vi "Tosca-Clear Trial Marker.vi"(11 "AODO":T1) -> (3 "AODO Out":T1)   [LabVIEW 2020]
uses:
  Typedefs/Tosca-State AODO.ctl
  epl-vi-lib/Signal Synthesis VIs/4th Generation/Classes/SignalManager/SignalManager.lvclass
  Typedefs/Tosca-AO Runtime.ctl
  Typedefs/Tosca-DO Runtime.ctl
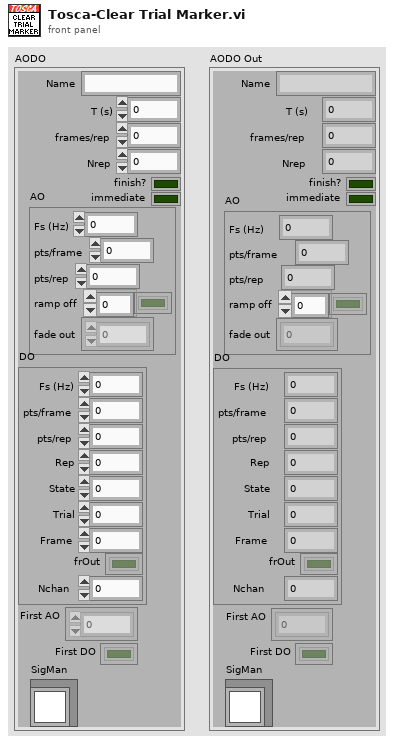
[diagram p1: front panel]
types:
  T1 = typedef "Tosca-State AODO.ctl" = cluster{"Name":string, "T (s)":dbl, "First AO":dbl[][], "frames/rep":i32, "finish?":bool, "Nrep":i32, "AO":T2, "DO":T3, "immediate":bool, "First DO":bool[][], "SigMan":refnum<class "SignalManager.lvclass">}
  T2 = typedef "Tosca-AO Runtime.ctl" = cluster{"Fs (Hz)":dbl, "pts/frame":i32, "pts/rep":i32, "ramp off":bool[], "fade out":dbl[][]}
  T3 = typedef "Tosca-DO Runtime.ctl" = cluster{"Fs (Hz)":dbl, "pts/frame":i32, "pts/rep":i32, "Rep":i32, "State":i32, "Trial":i32, "Frame":i32, "frOut":bool[], "Nchan":i32}
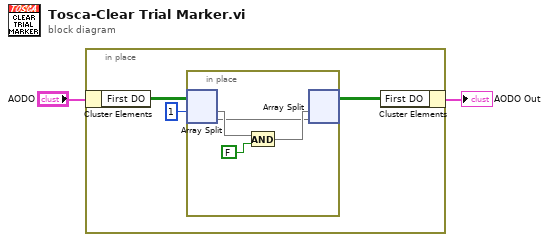
[diagram p0: block diagram]
diagram:
  n1 = in-place {
    n2 = in-place-cluster #1("AODO") -> ("First DO"=w5:bool[][])
    n3 = in-place {
      n4 = in-place-split #2(w5, 1) -> (w8:bool[][], w6:bool[][])
      n5 = And(x=w8, y=FALSE) -> (x .and. y?=w7:bool[][])
      n6 = in-place-split #2(w7, w6) -> (w4:bool[][])  [unwired: 1 out]
    }
    n7 = in-place-cluster #1("First DO"=w4) -> (→"AODO Out":T1)
  }
